vi "E6.vi"() -> ()   [LabVIEW 2017]
uses:
  <vilib>/userdefined/High Color/IMAQdx.ctl
  <vilib>/myRIO/Instrument Drivers/Onboard IO/DIO/typedefs/DIO Reference.ctl
  <vilib>/myRIO/Common/Instrument Driver Framework/Utilities/typedefs/myRIO Generic Hardware Reference.ctl
  <vilib>/myRIO/Common/Instrument Driver Framework/Utilities/typedefs/Hardware Version Enum.ctl
  <vilib>/myRIO/Common/Instrument Driver Framework/Utilities/typedefs/myRIO v1.0 Reference.ctl
  <vilib>/myRIO/Common/Instrument Driver Framework/Utilities/typedefs/Generic FPGA Reference.ctl
  <vilib>/myRIO/Common/Instrument Driver Framework/myRIO v1.0/DIO/typedefs/DIO Channels List.ctl
  <vilib>/myRIO/Common/Instrument Driver Framework/myRIO v1.0/DIO/typedefs/DIO Channels Enum.ctl
  <vilib>/userdefined/High Color/nirio_resource_hc.ctl
  <vilib>/myRIO/Common/Instrument Driver Framework/Utilities/vis/Is FPGA Ref Available.vi
  <vilib>/myRIO/Common/Instrument Driver Framework/myRIO v1.0/DIO/vis/myRIO v1.1 Open DIO.vi
  <vilib>/myRIO/Instrument Drivers/Onboard IO/DIO/vis/Write.vi
  <vilib>/myRIO/Common/Instrument Driver Framework/Utilities/vis/Validate Channels.vi
  <vilib>/myRIO/Common/Instrument Driver Framework/myRIO v1.0/DIO/vis/myRIO v1.0 Reserve DIO.vi
  <vilib>/myRIO/Common/Instrument Driver Framework/myRIO v1.0/Resource Manager/vis/myRIO v1.0 Reserve Channel List.vi
  <vilib>/myRIO/Common/Instrument Driver Framework/myRIO v1.0/DIO/vis/myRIO v1.0 Build MUX Configuration DIO.vi
  <vilib>/myRIO/Common/Instrument Driver Framework/myRIO v1.0/Resource Manager/vis/myRIO v1.0 Reserve Channel.vi
  <vilib>/myRIO/Common/Instrument Driver Framework/myRIO v1.0/Resource Manager/vis/myRIO v1.0 Unreserve Channel.vi
  <vilib>/myRIO/Common/Instrument Driver Framework/myRIO v1.0/Resource Manager/vis/myRIO v1.0 Create Configuration List.vi
  <vilib>/myRIO/Common/Instrument Driver Framework/myRIO v1.0/Resource Manager/vis/myRIO v1.0 Build Mutex Name.vi
  <vilib>/Utility/VariantDataType/GetNumericInfo.vi
  <vilib>/Utility/error.llb/Error Cluster From Error Code.vi
  <vilib>/myRIO/Common/Instrument Driver Framework/myRIO v1.0/myRIO v1.1 Open.vi
  <vilib>/myRIO/Common/Instrument Driver Framework/Utilities/vis/IO Manager.vi
  <vilib>/myRIO/Common/Instrument Driver Framework/Utilities/vis/Configuration Manager.vi
  <vilib>/myRIO/Common/Instrument Driver Framework/myRIO v1.0/Resource Manager/vis/myRIO v1.0 Configure IO.vi
  <vilib>/myRIO/Common/Instrument Driver Framework/myRIO v1.0/myRIO v1.0 Close.vi
  <vilib>/myRIO/Common/Instrument Driver Framework/myRIO v1.0/DIO/vis/myRIO v1.0 Write DIO.vi
  <vilib>/myRIO/Express VI/Onboard Devices/LED/LED Express VI.xnode
  <vilib>/myRIO/Instrument Drivers/Onboard IO/DIO/vis/myRIO DIO Open.xnode
  <vilib>/vision/driver/NI_Vision_Acquisition_Software.lvlib
  <vilib>/myRIO/Instrument Drivers/Onboard IO/DIO/DIO.lvlib
panel:
  out "лево":i32
  out "Image":T1(plugin-control)
  out "право":i32
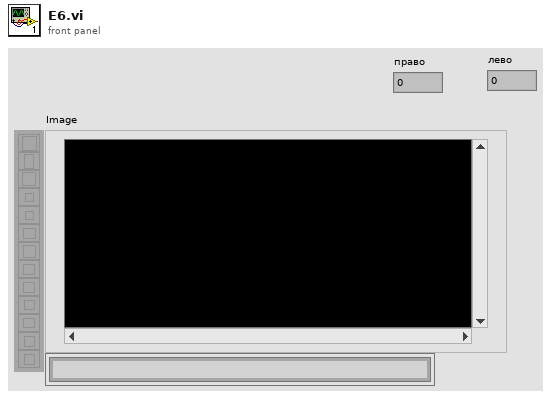
[diagram p1: front panel]
types:
  T1 = typedef "IMAQ Image.ctl" = refnum<image>
  T2 = typedef "IMAQdx.ctl" = refnum<k21>
  T3 = typedef "DIO.lvlib/DIO Reference.ctl" = cluster{"myRIO Reference":T4, "DIO Channels List":T8}
  T4 = typedef "myRIO Generic Hardware Reference.ctl" = cluster{"myRIO Model":T5, "myRIO Hardware Reference":T6}
  T5 = typedef "Hardware Version Enum.ctl" = enum16{"Unknown", "myRIO-1900", "myRIO-1950", "roboRIO", "NI ELVIS RIO CM"}
  T6 = typedef "myRIO v1.0 Reference.ctl" = cluster{"Generic FPGA Reference":T7, "Allow multiple opens":bool}
  T7 = typedef "Generic FPGA Reference.ctl" = refnum<k20>
  T8 = typedef "DIO Channels List.ctl" = T9[]
  T9 = typedef "DIO Channels Enum.ctl" = enum16{"Not Connected", "C/DIO0", "C/DIO1", "C/DIO2", "C/DIO3", "C/DIO4", "C/DIO5", "C/DIO6", "C/DIO7", "A/DIO0", "A/DIO1", "A/DIO2", "A/DIO3", "A/DIO4", "A/DIO5", "A/DIO6", "A/DIO7", "A/DIO8", "A/DIO9", "A/DIO10", "A/DIO11", "A/DIO12", "A/DIO13", "A/DIO14", "A/DIO15", "B/DIO0", "B/DIO1", "B/DIO2", "B/DIO3", "B/DIO4", "B/DIO5", "B/DIO6", "B/DIO7", "B/DIO8", "B/DIO9", "B/DIO10", "B/DIO11", "B/DIO12", "B/DIO13", "B/DIO14", "B/DIO15", "LED0", "LED1", "LED2", "LED3", "Button0", "DIO/DIO0", "DIO/DIO1", "DIO/DIO2", "DIO/DIO3", "DIO/DIO4", "DIO/DIO5", "DIO/DIO6", "DIO/DIO7", "DIO/DIO8", "DIO/DIO9", "SPI/CS0", "SPI/CS1", "SPI/CS2", "SPI/CS3", "LED RADIO (Green)", "LED RADIO (Red)", "LED COMM (Green)", "LED COMM (Red)", "LED MODE (Green)", "LED MODE (Red)"}
  T10 = typedef "nirio_resource_hc.ctl" = tag
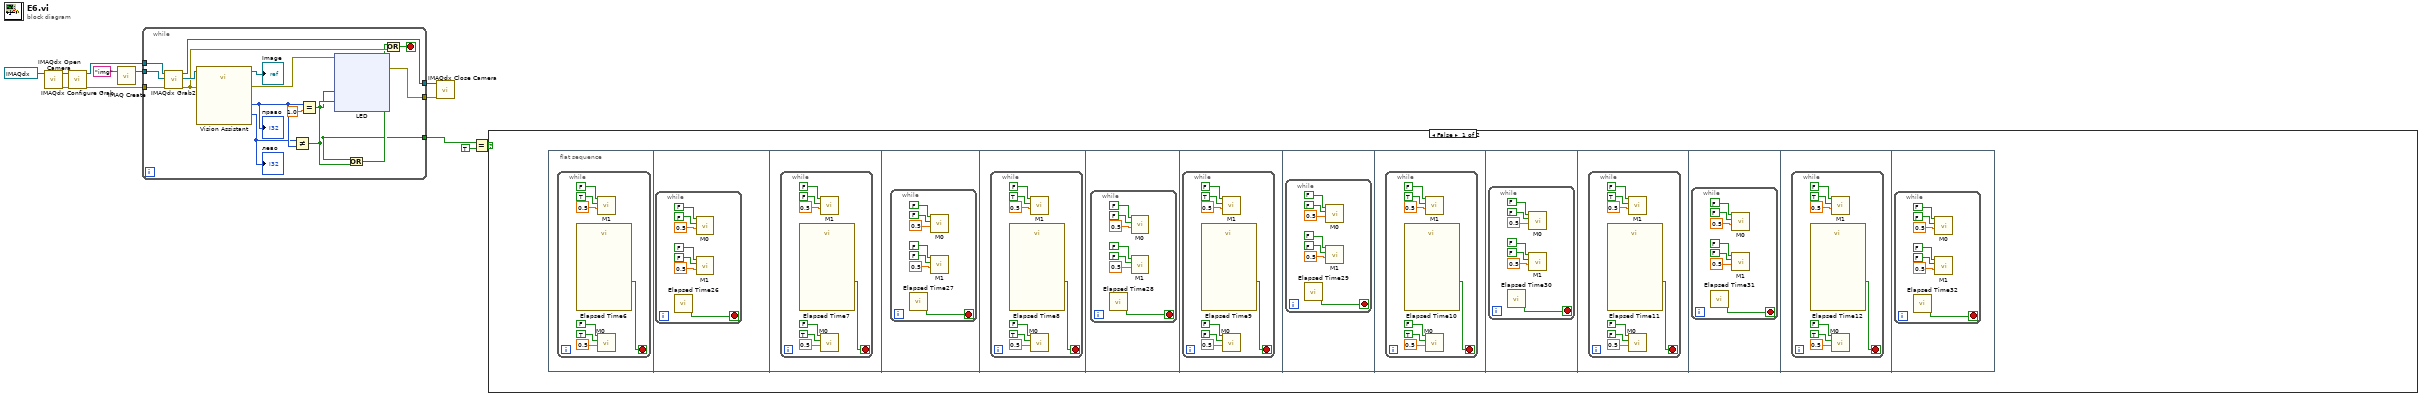
[diagram p0: block diagram]
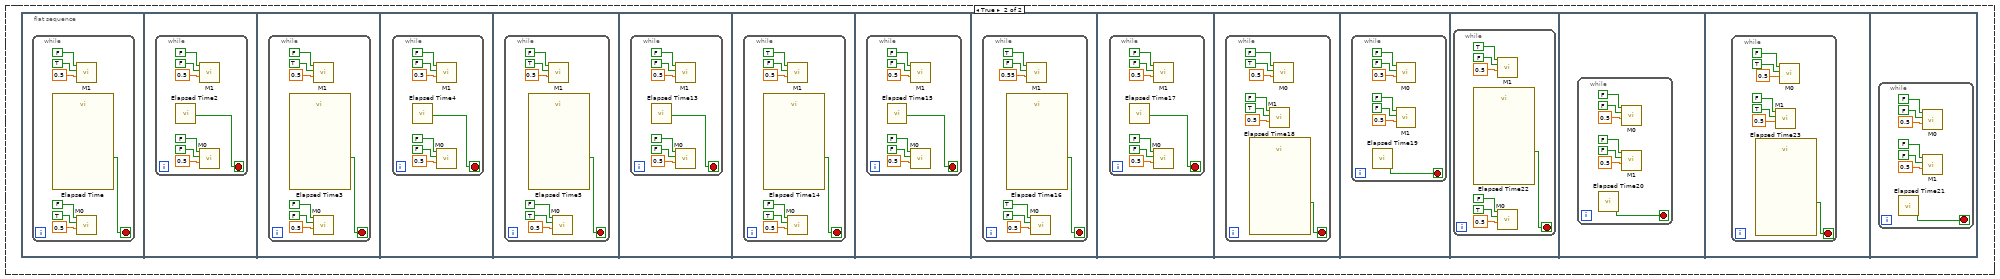
[diagram p2: hidden frame]
diagram:
  n1 = call <vilib>:"IMAQdx Open Camera.vi"("Session In"=T2 "cam0") -> ("error out"=w6:errorcluster, "Session Out"=w9:T2)  [unwired: 9 in]
  n2 = call <vilib>:"IMAQdx Configure Grab.vi"("error in"=w6, "Session In"=w9) -> ("error out"=w7:errorcluster, "Session Out"=w10:T2)  [unwired: 8 in]
  n3 = call "IMAQ Create"("Image Name"="img") -> ("New Image"=w8:T1)  [unwired: 4 in, 1 out]
  n4 = while {
    tunnel: w7 -> [w28]
    tunnel: w8 -> [w26]
    tunnel: w10 -> [w25]
    tunnel: [w24] -> w11
    tunnel: [w19] -> w12
    tunnel: [w13] -> w1
    stop <- w27 stop-if-true
    n5 = call <vilib>:"IMAQdx Grab2.vi"("error in"=w28, "Image In"=w26, "Session In"=w25) -> ("error out"=w21:errorcluster, "Image Out"=w22:T1, "Session Out"=w24:T2)  [unwired: 5 in, 1 out]
    n6 = call "Vision Assistant"("Image In"=w22, "error in"=w21) -> ("Image Out"=→"Image":T1, "Number of Matches (Pattern Matching 1)"=w16:i32, "Number of Matches (Pattern Matching 2)"=w15:i32, "error out"=w18:errorcluster)  [unwired: 22 in]
    "право" <- w16
    "лево" <- w15
    n7 = Not Equal?(x=w15, y=w16) -> (x != y?=w14:bool)
    n8 = Equal?(x=w16, y=1.0) -> (x = y?=w13:bool)
    n9 = xnode "LED"("LED1"=w13, "LED3"=w14, "error in (no error)"=w18) -> ("error out"=w19:errorcluster)
    n10 = Or(x=w13, y=w14) -> (x .or. y?=w17:bool)
    n11 = Or(x=w17, y=w21) -> (x .or. y?=w27:bool)
  }
  n12 = call <vilib>:"IMAQdx Close Camera.vi"("error in"=w12, "Session In"=w11) -> ()  [unwired: 9 in, 1 out]
  n13 = Equal?(x=w1, y=TRUE) -> (x = y?=w2:bool)
  n14 = case shown="False" w2 {
    frame False {
      n15 = flat-sequence {
        frame #0 {
          n16 = while {
            stop <- w65 stop-if-true
            n17 = call "Elapsed Time6"() -> ("Time has Elapsed"=w65:bool)  [unwired: 12 in, 7 out]
            n18 = call "M1.vi"("Duty Cycle"=0.5, "назад"=TRUE ("вперед"), "вперед"=FALSE ("назад")) -> ()  [unwired: 8 in, 1 out]
            n19 = call "M0.vi"("Duty Cycle"=0.5, "назад"=TRUE ("вперед"), "вперед"=FALSE ("назад")) -> ()  [unwired: 8 in, 1 out]
          }
        }
        frame #1 {
          n20 = while {
            stop <- w72 stop-if-true
            n21 = call "Elapsed Time26"() -> ("Time has Elapsed"=w72:bool)  [unwired: 12 in, 7 out]
            n22 = call "M0.vi"("Duty Cycle"=0.5, "назад"=FALSE ("вперед"), "вперед"=FALSE ("назад")) -> ()  [unwired: 8 in, 1 out]
            n23 = call "M1.vi"("Duty Cycle"=0.5, "назад"=FALSE ("вперед"), "вперед"=FALSE ("назад")) -> ()  [unwired: 8 in, 1 out]
          }
        }
        frame #2 {
          n24 = while {
            stop <- w79 stop-if-true
            n25 = call "Elapsed Time7"() -> ("Time has Elapsed"=w79:bool)  [unwired: 12 in, 7 out]
            n26 = call "M1.vi"("Duty Cycle"=0.5, "назад"=FALSE ("вперед"), "вперед"=FALSE ("назад")) -> ()  [unwired: 8 in, 1 out]
            n27 = call "M0.vi"("Duty Cycle"=0.5, "назад"=TRUE ("вперед"), "вперед"=FALSE ("назад")) -> ()  [unwired: 8 in, 1 out]
          }
        }
        frame #3 {
          n28 = while {
            stop <- w86 stop-if-true
            n29 = call "Elapsed Time27"() -> ("Time has Elapsed"=w86:bool)  [unwired: 12 in, 7 out]
            n30 = call "M0.vi"("Duty Cycle"=0.5, "назад"=FALSE ("вперед"), "вперед"=FALSE ("назад")) -> ()  [unwired: 8 in, 1 out]
            n31 = call "M1.vi"("Duty Cycle"=0.5, "назад"=FALSE ("вперед"), "вперед"=FALSE ("назад")) -> ()  [unwired: 8 in, 1 out]
          }
        }
        frame #4 {
          n32 = while {
            stop <- w93 stop-if-true
            n33 = call "Elapsed Time8"() -> ("Time has Elapsed"=w93:bool)  [unwired: 12 in, 7 out]
            n34 = call "M1.vi"("Duty Cycle"=0.5, "назад"=TRUE ("вперед"), "вперед"=FALSE ("назад")) -> ()  [unwired: 8 in, 1 out]
            n35 = call "M0.vi"("Duty Cycle"=0.5, "назад"=TRUE ("вперед"), "вперед"=FALSE ("назад")) -> ()  [unwired: 8 in, 1 out]
          }
        }
        frame #5 {
          n36 = while {
            stop <- w100 stop-if-true
            n37 = call "Elapsed Time28"() -> ("Time has Elapsed"=w100:bool)  [unwired: 12 in, 7 out]
            n38 = call "M0.vi"("Duty Cycle"=0.5, "назад"=FALSE ("вперед"), "вперед"=FALSE ("назад")) -> ()  [unwired: 8 in, 1 out]
            n39 = call "M1.vi"("Duty Cycle"=0.5, "назад"=FALSE ("вперед"), "вперед"=FALSE ("назад")) -> ()  [unwired: 8 in, 1 out]
          }
        }
        frame #6 {
          n40 = while {
            stop <- w107 stop-if-true
            n41 = call "Elapsed Time9"() -> ("Time has Elapsed"=w107:bool)  [unwired: 12 in, 7 out]
            n42 = call "M1.vi"("Duty Cycle"=0.5, "назад"=TRUE ("вперед"), "вперед"=FALSE ("назад")) -> ()  [unwired: 8 in, 1 out]
            n43 = call "M0.vi"("Duty Cycle"=0.5, "назад"=FALSE ("вперед"), "вперед"=FALSE ("назад")) -> ()  [unwired: 8 in, 1 out]
          }
        }
        frame #7 {
          n44 = while {
            stop <- w114 stop-if-true
            n45 = call "Elapsed Time29"() -> ("Time has Elapsed"=w114:bool)  [unwired: 12 in, 7 out]
            n46 = call "M0.vi"("Duty Cycle"=0.5, "назад"=FALSE ("вперед"), "вперед"=FALSE ("назад")) -> ()  [unwired: 8 in, 1 out]
            n47 = call "M1.vi"("Duty Cycle"=0.5, "назад"=FALSE ("вперед"), "вперед"=FALSE ("назад")) -> ()  [unwired: 8 in, 1 out]
          }
        }
        frame #8 {
          n48 = while {
            stop <- w121 stop-if-true
            n49 = call "Elapsed Time10"() -> ("Time has Elapsed"=w121:bool)  [unwired: 12 in, 7 out]
            n50 = call "M1.vi"("Duty Cycle"=0.5, "назад"=TRUE ("вперед"), "вперед"=FALSE ("назад")) -> ()  [unwired: 8 in, 1 out]
            n51 = call "M0.vi"("Duty Cycle"=0.5, "назад"=TRUE ("вперед"), "вперед"=FALSE ("назад")) -> ()  [unwired: 8 in, 1 out]
          }
        }
        frame #9 {
          n52 = while {
            stop <- w128 stop-if-true
            n53 = call "Elapsed Time30"() -> ("Time has Elapsed"=w128:bool)  [unwired: 12 in, 7 out]
            n54 = call "M0.vi"("Duty Cycle"=0.5, "назад"=FALSE ("вперед"), "вперед"=FALSE ("назад")) -> ()  [unwired: 8 in, 1 out]
            n55 = call "M1.vi"("Duty Cycle"=0.5, "назад"=FALSE ("вперед"), "вперед"=FALSE ("назад")) -> ()  [unwired: 8 in, 1 out]
          }
        }
        frame #10 {
          n56 = while {
            stop <- w135 stop-if-true
            n57 = call "Elapsed Time11"() -> ("Time has Elapsed"=w135:bool)  [unwired: 12 in, 7 out]
            n58 = call "M1.vi"("Duty Cycle"=0.5, "назад"=TRUE ("вперед"), "вперед"=FALSE ("назад")) -> ()  [unwired: 8 in, 1 out]
            n59 = call "M0.vi"("Duty Cycle"=0.5, "назад"=FALSE ("вперед"), "вперед"=FALSE ("назад")) -> ()  [unwired: 8 in, 1 out]
          }
        }
        frame #11 {
          n60 = while {
            stop <- w142 stop-if-true
            n61 = call "Elapsed Time31"() -> ("Time has Elapsed"=w142:bool)  [unwired: 12 in, 7 out]
            n62 = call "M0.vi"("Duty Cycle"=0.5, "назад"=FALSE ("вперед"), "вперед"=FALSE ("назад")) -> ()  [unwired: 8 in, 1 out]
            n63 = call "M1.vi"("Duty Cycle"=0.5, "назад"=FALSE ("вперед"), "вперед"=FALSE ("назад")) -> ()  [unwired: 8 in, 1 out]
          }
        }
        frame #12 {
          n64 = while {
            stop <- w149 stop-if-true
            n65 = call "Elapsed Time12"() -> ("Time has Elapsed"=w149:bool)  [unwired: 12 in, 7 out]
            n66 = call "M1.vi"("Duty Cycle"=0.5, "назад"=TRUE ("вперед"), "вперед"=FALSE ("назад")) -> ()  [unwired: 8 in, 1 out]
            n67 = call "M0.vi"("Duty Cycle"=0.5, "назад"=TRUE ("вперед"), "вперед"=FALSE ("назад")) -> ()  [unwired: 8 in, 1 out]
          }
        }
        frame #13 {
          n68 = while {
            stop <- w156 stop-if-true
            n69 = call "Elapsed Time32"() -> ("Time has Elapsed"=w156:bool)  [unwired: 12 in, 7 out]
            n70 = call "M0.vi"("Duty Cycle"=0.5, "назад"=FALSE ("вперед"), "вперед"=FALSE ("назад")) -> ()  [unwired: 8 in, 1 out]
            n71 = call "M1.vi"("Duty Cycle"=0.5, "назад"=FALSE ("вперед"), "вперед"=FALSE ("назад")) -> ()  [unwired: 8 in, 1 out]
          }
        }
      }
    }
    frame True {
      n72 = flat-sequence {
        frame #0 {
          n73 = while {
            stop <- w163 stop-if-true
            n74 = call "Elapsed Time"() -> ("Time has Elapsed"=w163:bool)  [unwired: 12 in, 7 out]
            n75 = call "M1.vi"("Duty Cycle"=0.5, "назад"=TRUE ("вперед"), "вперед"=FALSE ("назад")) -> ()  [unwired: 8 in, 1 out]
            n76 = call "M0.vi"("Duty Cycle"=0.5, "назад"=TRUE ("вперед"), "вперед"=FALSE ("назад")) -> ()  [unwired: 8 in, 1 out]
          }
        }
        frame #1 {
          n77 = while {
            stop <- w170 stop-if-true
            n78 = call "Elapsed Time2"() -> ("Time has Elapsed"=w170:bool)  [unwired: 12 in, 7 out]
            n79 = call "M1.vi"("Duty Cycle"=0.5, "назад"=FALSE ("вперед"), "вперед"=FALSE ("назад")) -> ()  [unwired: 8 in, 1 out]
            n80 = call "M0.vi"("Duty Cycle"=0.5, "назад"=FALSE ("вперед"), "вперед"=FALSE ("назад")) -> ()  [unwired: 8 in, 1 out]
          }
        }
        frame #2 {
          n81 = while {
            stop <- w177 stop-if-true
            n82 = call "Elapsed Time3"() -> ("Time has Elapsed"=w177:bool)  [unwired: 12 in, 7 out]
            n83 = call "M1.vi"("Duty Cycle"=0.5, "назад"=TRUE ("вперед"), "вперед"=FALSE ("назад")) -> ()  [unwired: 8 in, 1 out]
            n84 = call "M0.vi"("Duty Cycle"=0.5, "назад"=FALSE ("вперед"), "вперед"=FALSE ("назад")) -> ()  [unwired: 8 in, 1 out]
          }
        }
        frame #3 {
          n85 = while {
            stop <- w184 stop-if-true
            n86 = call "Elapsed Time4"() -> ("Time has Elapsed"=w184:bool)  [unwired: 12 in, 7 out]
            n87 = call "M1.vi"("Duty Cycle"=0.5, "назад"=FALSE ("вперед"), "вперед"=FALSE ("назад")) -> ()  [unwired: 8 in, 1 out]
            n88 = call "M0.vi"("Duty Cycle"=0.5, "назад"=FALSE ("вперед"), "вперед"=FALSE ("назад")) -> ()  [unwired: 8 in, 1 out]
          }
        }
        frame #4 {
          n89 = while {
            stop <- w191 stop-if-true
            n90 = call "Elapsed Time5"() -> ("Time has Elapsed"=w191:bool)  [unwired: 12 in, 7 out]
            n91 = call "M1.vi"("Duty Cycle"=0.5, "назад"=TRUE ("вперед"), "вперед"=FALSE ("назад")) -> ()  [unwired: 8 in, 1 out]
            n92 = call "M0.vi"("Duty Cycle"=0.5, "назад"=TRUE ("вперед"), "вперед"=FALSE ("назад")) -> ()  [unwired: 8 in, 1 out]
          }
        }
        frame #5 {
          n93 = while {
            stop <- w198 stop-if-true
            n94 = call "Elapsed Time13"() -> ("Time has Elapsed"=w198:bool)  [unwired: 12 in, 7 out]
            n95 = call "M1.vi"("Duty Cycle"=0.5, "назад"=FALSE ("вперед"), "вперед"=FALSE ("назад")) -> ()  [unwired: 8 in, 1 out]
            n96 = call "M0.vi"("Duty Cycle"=0.5, "назад"=FALSE ("вперед"), "вперед"=FALSE ("назад")) -> ()  [unwired: 8 in, 1 out]
          }
        }
        frame #6 {
          n97 = while {
            stop <- w205 stop-if-true
            n98 = call "Elapsed Time14"() -> ("Time has Elapsed"=w205:bool)  [unwired: 12 in, 7 out]
            n99 = call "M1.vi"("Duty Cycle"=0.5, "назад"=FALSE ("вперед"), "вперед"=TRUE ("назад")) -> ()  [unwired: 8 in, 1 out]
            n100 = call "M0.vi"("Duty Cycle"=0.5, "назад"=TRUE ("вперед"), "вперед"=FALSE ("назад")) -> ()  [unwired: 8 in, 1 out]
          }
        }
        frame #7 {
          n101 = while {
            stop <- w212 stop-if-true
            n102 = call "Elapsed Time15"() -> ("Time has Elapsed"=w212:bool)  [unwired: 12 in, 7 out]
            n103 = call "M1.vi"("Duty Cycle"=0.5, "назад"=FALSE ("вперед"), "вперед"=FALSE ("назад")) -> ()  [unwired: 8 in, 1 out]
            n104 = call "M0.vi"("Duty Cycle"=0.5, "назад"=FALSE ("вперед"), "вперед"=FALSE ("назад")) -> ()  [unwired: 8 in, 1 out]
          }
        }
        frame #8 {
          n105 = while {
            stop <- w219 stop-if-true
            n106 = call "Elapsed Time16"() -> ("Time has Elapsed"=w219:bool)  [unwired: 12 in, 7 out]
            n107 = call "M1.vi"("Duty Cycle"=0.55, "назад"=FALSE ("вперед"), "вперед"=TRUE ("назад")) -> ()  [unwired: 8 in, 1 out]
            n108 = call "M0.vi"("Duty Cycle"=0.5, "назад"=FALSE ("вперед"), "вперед"=TRUE ("назад")) -> ()  [unwired: 8 in, 1 out]
          }
        }
        frame #9 {
          n109 = while {
            stop <- w226 stop-if-true
            n110 = call "Elapsed Time17"() -> ("Time has Elapsed"=w226:bool)  [unwired: 12 in, 7 out]
            n111 = call "M1.vi"("Duty Cycle"=0.5, "назад"=FALSE ("вперед"), "вперед"=FALSE ("назад")) -> ()  [unwired: 8 in, 1 out]
            n112 = call "M0.vi"("Duty Cycle"=0.5, "назад"=FALSE ("вперед"), "вперед"=FALSE ("назад")) -> ()  [unwired: 8 in, 1 out]
          }
        }
        frame #10 {
          n113 = while {
            stop <- w233 stop-if-true
            n114 = call "Elapsed Time18"() -> ("Time has Elapsed"=w233:bool)  [unwired: 12 in, 7 out]
            n115 = call "M1.vi"("Duty Cycle"=0.5, "назад"=TRUE ("вперед"), "вперед"=FALSE ("назад")) -> ()  [unwired: 8 in, 1 out]
            n116 = call "M0.vi"("Duty Cycle"=0.5, "назад"=TRUE ("вперед"), "вперед"=FALSE ("назад")) -> ()  [unwired: 8 in, 1 out]
          }
        }
        frame #11 {
          n117 = while {
            stop <- w240 stop-if-true
            n118 = call "Elapsed Time19"() -> ("Time has Elapsed"=w240:bool)  [unwired: 12 in, 7 out]
            n119 = call "M0.vi"("Duty Cycle"=0.5, "назад"=FALSE ("вперед"), "вперед"=FALSE ("назад")) -> ()  [unwired: 8 in, 1 out]
            n120 = call "M1.vi"("Duty Cycle"=0.5, "назад"=FALSE ("вперед"), "вперед"=FALSE ("назад")) -> ()  [unwired: 8 in, 1 out]
          }
        }
        frame #12 {
          n121 = while {
            stop <- w247 stop-if-true
            n122 = call "Elapsed Time22"() -> ("Time has Elapsed"=w247:bool)  [unwired: 12 in, 7 out]
            n123 = call "M1.vi"("Duty Cycle"=0.5, "назад"=FALSE ("вперед"), "вперед"=TRUE ("назад")) -> ()  [unwired: 8 in, 1 out]
            n124 = call "M0.vi"("Duty Cycle"=0.5, "назад"=TRUE ("вперед"), "вперед"=FALSE ("назад")) -> ()  [unwired: 8 in, 1 out]
          }
        }
        frame #13 {
          n125 = while {
            stop <- w254 stop-if-true
            n126 = call "Elapsed Time20"() -> ("Time has Elapsed"=w254:bool)  [unwired: 12 in, 7 out]
            n127 = call "M0.vi"("Duty Cycle"=0.5, "назад"=FALSE ("вперед"), "вперед"=FALSE ("назад")) -> ()  [unwired: 8 in, 1 out]
            n128 = call "M1.vi"("Duty Cycle"=0.5, "назад"=FALSE ("вперед"), "вперед"=FALSE ("назад")) -> ()  [unwired: 8 in, 1 out]
          }
        }
        frame #14 {
          n129 = while {
            stop <- w261 stop-if-true
            n130 = call "Elapsed Time23"() -> ("Time has Elapsed"=w261:bool)  [unwired: 12 in, 7 out]
            n131 = call "M1.vi"("Duty Cycle"=0.5, "назад"=TRUE ("вперед"), "вперед"=FALSE ("назад")) -> ()  [unwired: 8 in, 1 out]
            n132 = call "M0.vi"("Duty Cycle"=0.5, "назад"=TRUE ("вперед"), "вперед"=FALSE ("назад")) -> ()  [unwired: 8 in, 1 out]
          }
        }
        frame #15 {
          n133 = while {
            stop <- w268 stop-if-true
            n134 = call "Elapsed Time21"() -> ("Time has Elapsed"=w268:bool)  [unwired: 12 in, 7 out]
            n135 = call "M0.vi"("Duty Cycle"=0.5, "назад"=FALSE ("вперед"), "вперед"=FALSE ("назад")) -> ()  [unwired: 8 in, 1 out]
            n136 = call "M1.vi"("Duty Cycle"=0.5, "назад"=FALSE ("вперед"), "вперед"=FALSE ("назад")) -> ()  [unwired: 8 in, 1 out]
          }
        }
      }
    }
  }
